vi "ScanFloatFromString.vi"(8 "errorIn":errorcluster, 11 "String":string) -> (0 "error Out":errorcluster, 3 "Float":dbl)   [LabVIEW 2009]
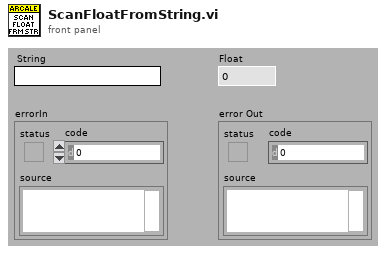
[diagram p1: front panel]
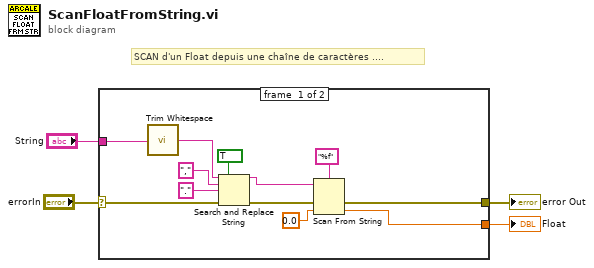
[diagram p0: block diagram]
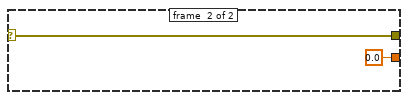
[diagram p2: hidden frame]
diagram:
  # "SCAN d'un Float depuis une chaîne de caractères ...."
  n1 = case shown="No Error" "errorIn" {
    selector: "errorIn" -> [w5 w18]
    tunnel: [w16 w18] -> w4
    tunnel: [w15 0.0 ("default value 1")] -> w3
    tunnel: "String" -> [w6 _]
    frame #0 {
      n2 = call <vilib>:"Trim Whitespace.vi"("string"=w6) -> ("trimmed string"=w7:string)  [unwired: 1 in]
      n3 = Search and Replace String(replace all?=TRUE ("replace all? (F)"), input string=w7, search string=",", replace string="." ("replace string (\"\")"), error in=w5) -> (result string=w12:string, error out=w11:errorcluster)  [unwired: 3 in, 2 out]
      n4 = Scan From String(format string="%f", input string=w12, error in=w11, default 1=0.0 ("default value 1")) -> (error out=w16:errorcluster, output 1=w15:dbl)  [unwired: 1 in, 2 out]
    }
    frame #1 {
    }
  }
  "error Out" <- w4
  "Float" <- w3
